vi "TEMPLATE.vi"(6 "Sender":refnum<class "Sender.lvclass">, 11 "TEMPLATE in":refnum<class "TEMPLATE.lvclass">) -> (0 "Error out":errorcluster, 3 "TEMPLATE out":refnum<class "TEMPLATE.lvclass">)   [LabVIEW 2025, in "_Template.lvlib" / "Templates.lvlib" / "TEMPLATE Msg.lvlib" / "TEMPLATE.lvclass"]
uses:
  TEMPLATE.lvclass
  jettl/jettl/Sender/Sender/Sender.lvclass
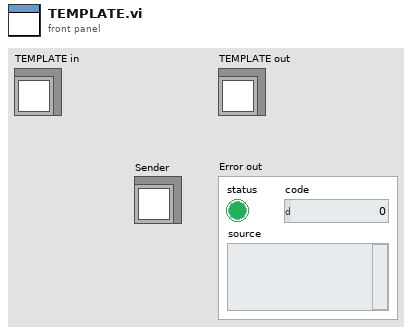
[diagram p1: front panel]
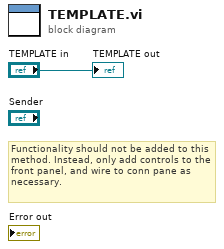
[diagram p0: block diagram]
diagram:
  # "Functionality should not be added to this method. Instead, only add controls to the front panel, and wire to conn pane as necessary."
  "TEMPLATE out" <- "TEMPLATE in"
